vi "server.vi"() -> ()   [LabVIEW 2020]
uses:
  <vilib>/Platform/TimedLoop/XDataNode/timing_clust.ctl
  <vilib>/Platform/TimedLoop/XDataNode/nitl_modes.ctl
  <vilib>/Platform/TimedLoop/XDataNode/wakeup.ctl
  <vilib>/platform/TimedLoop/XDataNode/XDataNode.xnode
  <vilib>/Platform/TimedLoop/XDataNode/XDNodeRunTimeDep.lvlib
panel:
  in  "vi path II":path=path "C:/Users/Sergey Denisov/Documents/REPS/TRANCON/test/hardware2.vi"
  in  "vi path I":path=path "C:/Users/Sergey Denisov/Documents/REPS/TRANCON/test/hardware1.vi"
  out "Numeric":i32
  in  "stop":bool
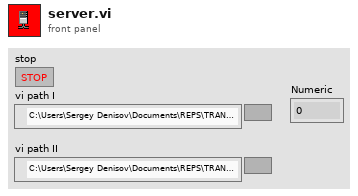
[diagram p1: front panel]
types:
  T1 = typedef "XDNodeRunTimeDep.lvlib/timing_clust.ctl" = cluster{"Expected End [f-1]":u64, "Actual End [f-1]":u64, "Finished Late? [f-1]":bool, "Expected End [i-1]":u64, "Actual End [i-1]":u64, "Finished Late? [i-1]":bool, "Expected Start [i]":u64, "Actual Start [i]":u64, "Expected Start [f]":u64, "Actual Start [f]":u64, "Source Name":string, "Structure Name":string, "Period":i64, "Deadline":i64, "Offset":i64, "Start":i64, "Priority":i32, "Timeout":i32, "Mode":T2, "Wakeup Reason":T3, "Error":errorcluster, "Source Type":string, "Secondary Source Type":string, "Global End Time":u64, "Global Start Time":u64, "Frame Duration":u64, "Iteration Duration":u64, "Assigned CPU":i32, "I/O Scan Engine Mode":u32}
  T2 = typedef "XDNodeRunTimeDep.lvlib/nitl_modes.ctl" = enum32{"No Change", "Process missed periods, maintain original phase", "Discard missed periods, maintain original phase", "Process missed periods, ignore original phase", "Discard missed periods, ignore original phase"}
  T3 = typedef "XDNodeRunTimeDep.lvlib/wakeup.ctl" = enum32{"Normal", "Aborted", "Asynchronous wakeup", "Timing source error", "Timed loop error", "Timeout"}
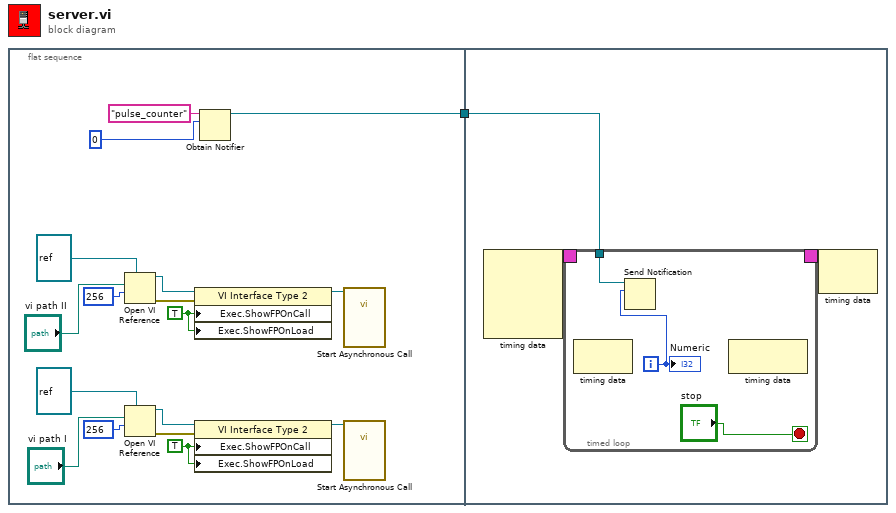
[diagram p0: block diagram]
diagram:
  n1 = flat-sequence {
    tunnel: [w2] -> w1
    tunnel: w1 -> [w19]
    frame #0 {
      w8 = TRUE ("Exécution:Afficher la face-avant à l'appel")
      w15 = TRUE ("Exécution:Afficher la face-avant à l'appel")
      n2 = Open VI Reference(type specifier VI Refnum (for type only)=refnum<vi> refnum ("spécificateur de type du refnum de VI (pour type seulement)"), vi path="vi path II", options=256) -> (vi reference=w6:refnum<vi>, error out=w7:errorcluster)  [unwired: 3 in]
      n3 = Open VI Reference(type specifier VI Refnum (for type only)=refnum<vi> refnum ("spécificateur de type du refnum de VI (pour type seulement)"), vi path="vi path I", options=256) -> (vi reference=w17:refnum<vi>, error out=w16:errorcluster)  [unwired: 3 in]
      n4 = property class="VI Interface Type 2"(reference=w6, error in=w7, "Exec.ShowFPOnCall"=w8, "Exec.ShowFPOnLoad"=w8) -> (reference out=w10:refnum<vi>)  [unwired: 1 out]
      n5 = property class="VI Interface Type 2"(reference=w17, error in=w16, "Exec.ShowFPOnCall"=w15, "Exec.ShowFPOnLoad"=w15) -> (reference out=w13:refnum<vi>)  [unwired: 1 out]
      n6 = Obtain Notifier(name (unnamed)="pulse_counter", notification data type=0) -> (notifier out=w2:refnum<notifier>)  [unwired: 2 in, 2 out]
      n7 = call-by-ref "Start Asynchronous Call"(reference=w10) -> ()  [unwired: 13 in, 2 out]
      n8 = call-by-ref "Start Asynchronous Call"(reference=w13) -> ()  [unwired: 13 in, 2 out]
    }
    frame #1 {
      n9 = node-c288() -> (w21:T1)  [unwired: 4 in]
      n10 = timed-loop {
        timing: w21 -> [_]
        timing-out: [_] -> w20
        tunnel: w19 -> [w23]
        i -> [w22]
        stop <- "stop" stop-if-true
        n11 = node-c288() -> ()  [unwired: 1 in, 1 out]
        n12 = Send Notification(notification=w22, notifier=w23) -> ()  [unwired: 1 in, 2 out]
        n13 = node-c288() -> ()  [unwired: 1 in, 1 out]
        "Numeric" <- w22
      }
      n14 = node-c288(w20) -> ()  [unwired: 1 out]
    }
  }
